vi "Sector Parameter Global.vi"() -> ()   [LabVIEW 2013]
uses:
  Sector/Accumulate/Sector Parameter Cluster.ctl
panel:
  out "Left - Right Cycle Output":fxp<+,8,0>
  out "Right Duty Cycle Output":fxp<+,8,0>
  out "Left Duty Cycle Output":fxp<+,8,0>
  in  "Right Start Angle Duty Cycle":fxp<+,8,0>
  in  "Right End Angle Duty Cycle":fxp<+,8,0>
  in  "Left End Angle Duty Cycle":fxp<+,8,0>
  in  "Left Start Angle Duty Cycle":fxp<+,8,0>
  in  "Sector Threshold":u8
  in  "[Average BG Intensity]":u8[](array[numeric])=[0, 0, 0, 0, 0, 0, 0, 0, 0, 0, 0, 0, 0, 0, 0, 0, 0, 0, 0, 0, 0, 0, 0, 0, 0, 0, 0, 0, 0, 0, 0, 0]
  in  "Sector Parameters Right":T1
  in  "Sector Parameters Left":T1
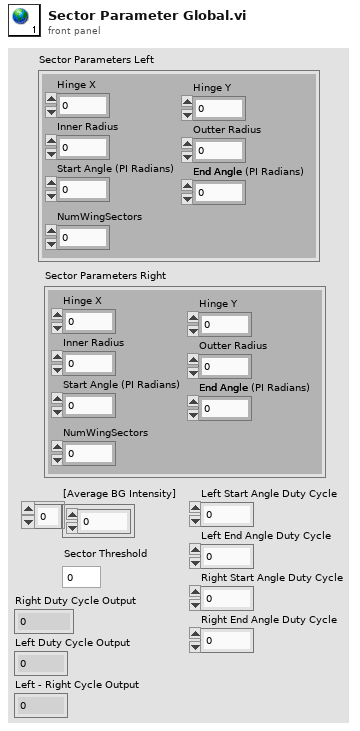
[diagram p1: front panel]
types:
  T1 = typedef "Sector Parameter Cluster.ctl" = cluster{"Start Angle":fxp<+/-,17,2>, "End Angle":fxp<+/-,17,2>, "Inner Radius":u16, "Outter Radius":u16, "Hinge X":u16, "Hinge Y":u16, "NumWingSectors":u8}
diagram:
